vi "Alumina Material Properties.vi"(6 "m-nm Al2O3":dbl, 9 "Alumina Thickness":dbl, 10 "Energy (Heat; I^2R)":dbl, 11 "NS Base Area":dbl) -> (1 "Volume Al2O3":dbl, 2 "Delta Temp Change Al2O3":dbl, 3 "Mass Al2O3":dbl, 4 "Al2O3 Thickness":dbl, 5 "Al2O3 Specfic Heat Capacity":dbl, 7 "Al2O3 Density":dbl, 8 "mc":dbl)   [LabVIEW 2020]
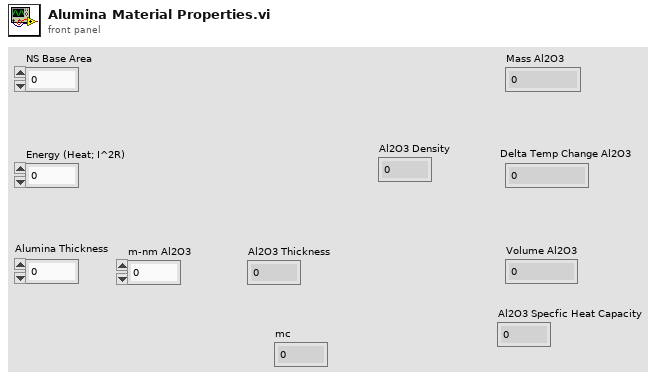
[diagram p1: front panel]
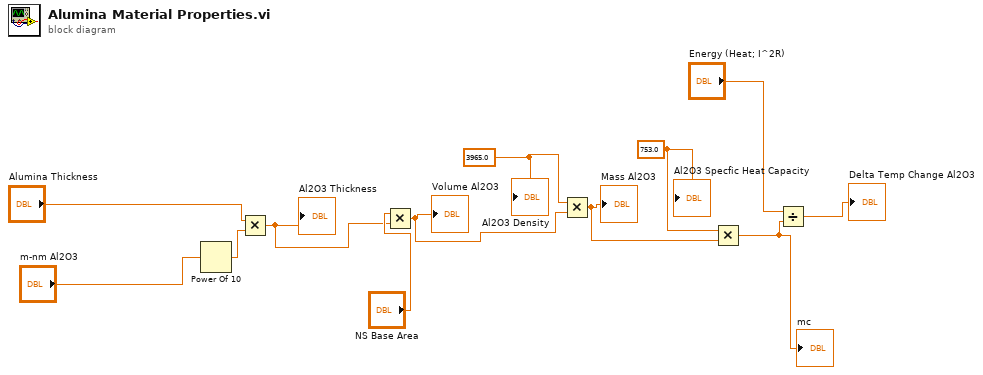
[diagram p0: block diagram]
diagram:
  w12 = 753.0 ("Silicon Specfic Heat Capacity 4")
  w7 = 3965.0 ("Silicon Density 4")
  n1 = Power Of 10(x="m-nm Al2O3") -> (10^x=w2:dbl)
  n2 = Multiply(x="Alumina Thickness", y=w2) -> (x*y=w5:dbl)
  "Al2O3 Thickness" <- w5
  n3 = Multiply(x="NS Base Area", y=w5) -> (x*y=w6:dbl)
  "Volume Al2O3" <- w6
  n4 = Multiply(x=w7, y=w6) -> (x*y=w11:dbl)
  "Mass Al2O3" <- w11
  n5 = Multiply(x=w12, y=w11) -> (x*y=w1:dbl)
  "mc" <- w1
  n6 = Divide(x="Energy (Heat; I^2R)", y=w1) -> (x/y=→"Delta Temp Change Al2O3":dbl)
  "Al2O3 Density" <- w7
  "Al2O3 Specfic Heat Capacity" <- w12
